vi "ADIS16470 IMU Example.vi"() -> ()   [LabVIEW 2019]
uses:
  <vilib>/Utility/RT CPU Load.ctl
  ADIS16470Lib/Typedef/ADIS16470 Hardware Configuration.ctl
  <vilib>/Rock Robotics/WPI/SPI/WPI_SPIMode.ctl
  <vilib>/Rock Robotics/SystemInterfaces/DIO/FPGA_DIOChannel.ctl
  <vilib>/Rock Robotics/SystemInterfaces/spilib/spi_bus.ctl
  <vilib>/NI_Real-Time Target Support.lvlib
panel:
  in  "Reset?":bool
  out "Integrated Gyro Angle":T1(graph)
  out "Calibrated?":bool
  out "Ready?":bool
  in  "Hardware Config":T2={"SPI Clock Rate (Hz)"=2000000.0, "IMU SPI Mode (3)"=enum."Mode 3 (Clk Idle High,Sample on Trailing)", "IMU Reset Pin"=enum."SPI Port CS2", "IMU SPI Bus"=enum."SPI On-Board, CS0", "IMU Data Ready Pin"=enum."SPI Port CS1", "Stall Config"={"Pow2BytesPerRead"=1, "StallTicks"=1000, "CsToSclkTicks"=5}}
  out "CPU loads":T6[](array[typedef]) {"ISR (%)" format="%#.2f"; "Idle (%)" format="%#.2f"; "Background (%)" format="%#.2f"; "Normal (%)" format="%#.2f"; "Above Normal (%)" format="%#.2f"; "High (%)" format="%#.2g"; "Timed Structures (%)" format="%#.2g"; "Time Critical (%)" format="%#.2g"; "Total (%)" format="%#.2g"}
  in  "stop":bool
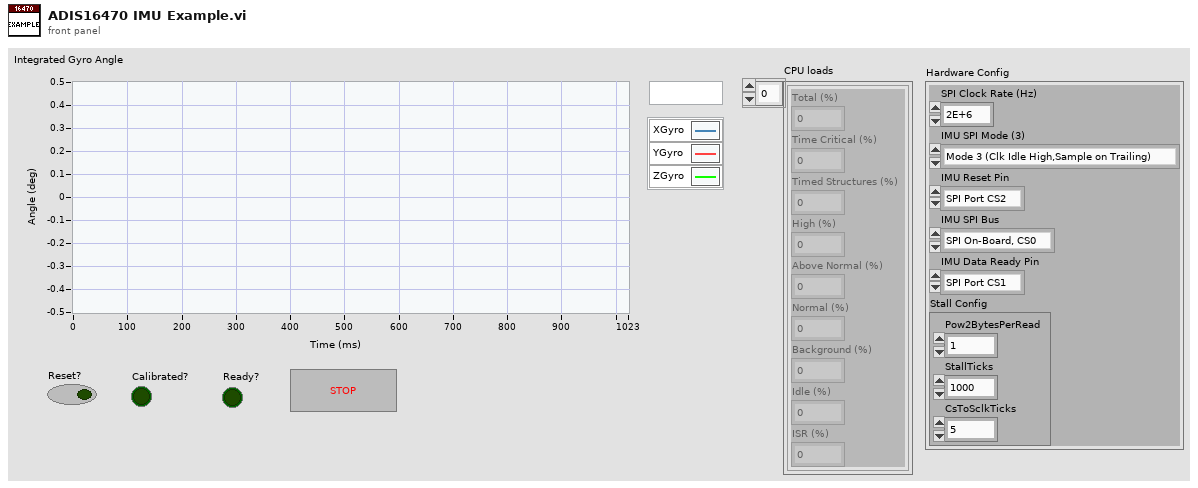
[diagram p1: front panel]
types:
  T1 = cluster{"XAngle":dbl, "YAngle":dbl, "ZAngle":dbl}
  T2 = typedef "ADIS16470 Hardware Configuration.ctl" = cluster{"SPI Clock Rate (Hz)":dbl, "IMU SPI Mode (3)":T3, "IMU Reset Pin":T4, "IMU SPI Bus":T5, "IMU Data Ready Pin":T4, "Stall Config":cluster{"Pow2BytesPerRead":u8, "StallTicks":u16, "CsToSclkTicks":u8}}
  T3 = typedef "WPI_SPIMode.ctl" = enum16{"Mode 0 (Clk Idle Low,Sample on Leading)", "Mode 1 (Clk Idle Low,Sample on Trailing)", "Mode 2 (Clk Idle High,Sample on Leading)", "Mode 3 (Clk Idle High,Sample on Trailing)"}
  T4 = typedef "FPGA_DIOChannel.ctl" = enum8{"DIO 0", "DIO 1", "DIO 2", "DIO 3", "DIO 4", "DIO 5", "DIO 6", "DIO 7", "DIO 8", "DIO 9", "DIO MXP 0", "DIO MXP 1", "DIO MXP 2", "DIO MXP 3", "DIO MXP 4", "DIO MXP 5", "DIO MXP 6", "DIO MXP 7", "DIO MXP 8", "DIO MXP 9", "DIO MXP 10", "DIO MXP 11", "DIO MXP 12", "DIO MXP 13", "DIO MXP 14", "DIO MXP 15", "SPI Port CS1", "SPI Port CS2", "SPI Port CS3", "SPI Port MISO", "SPI Port MOSI", "Invalid"}
  T5 = typedef "spi_bus.ctl" = enum16{"SPI On-Board, CS0", "SPI On-Board, CS1", "SPI On-Board, CS2", "SPI On-Board, CS3", "SPI MXP", "Invalid"}
  T6 = typedef "NI_Real-Time Target Support.lvlib/RT CPU Load.ctl" = cluster{"Total (%)":dbl, "Time Critical (%)":dbl, "Timed Structures (%)":dbl, "High (%)":dbl, "Above Normal (%)":dbl, "Normal (%)":dbl, "Background (%)":dbl, "Idle (%)":dbl, "ISR (%)":dbl}
  T7 = typedef "ADIS16470 Device Reference.ctl" = cluster{"DevStatus":errorcluster, "Hardware Config":T2, "End Calibration":refnum<notifier>, "Calibration Complete":refnum<notifier>, "Status FIFO":refnum<k33>, "Last Value Reference":refnum<data-value>, "Sychronous Process VI":T8, "Cmd FIFO":refnum<k33>, "Source":T9, "Data FIFO":refnum<k33>}
  T8 = typedef "ADIS16470 Process.ctl" = refnum<vi>
  T9 = typedef "FPGA_CounterEncoderSourceConvertionLVSourceType.ctl" = cluster{"DevStatus":errorcluster, "AnalogTriggerMode?":bool, "DigitalMode":cluster{"DIO Channel":T10}, "AnalogTriggerMode":cluster{"AnalogTriggerIndex":T11, "OutputType":T12}}
  T10 = typedef "FPGA_DIODigitalSourceChannel.ctl" = enum8{"DIO 0", "DIO 1", "DIO 2", "DIO 3", "DIO 4", "DIO 5", "DIO 6", "DIO 7", "DIO 8", "DIO 9", "DIO MXP 0", "DIO MXP 1", "DIO MXP 2", "DIO MXP 3", "DIO MXP 4", "DIO MXP 5", "DIO MXP 6", "DIO MXP 7", "DIO MXP 8", "DIO MXP 9", "DIO MXP 10", "DIO MXP 11", "DIO MXP 12", "DIO MXP 13", "DIO MXP 14", "DIO MXP 15", "SPI Port CS1", "SPI Port CS2", "SPI Port CS3", "SPI Port MISO", "SPI Port MOSI", "Disabled"}
  T11 = typedef "FPGA_AnalogTriggerIndex.ctl" = enum8{"Trig 0", "Trig 1", "Trig 2", "Trig 3", "Trig 4", "Trig 5", "Trig 6", "Trig 7", "Invalid"}
  T12 = typedef "FPGA_AnalogTriggerOutType.ctl" = enum16{"InWindow", "TriggerState", "Rising", "Falling"}
  T13 = typedef "ADIS16470 Status.ctl" = cluster{"Calibrated?":bool}
  T14 = typedef "ADIS16470 Data.ctl" = cluster{"XAngle":dbl, "YAngle":dbl, "ZAngle":dbl}
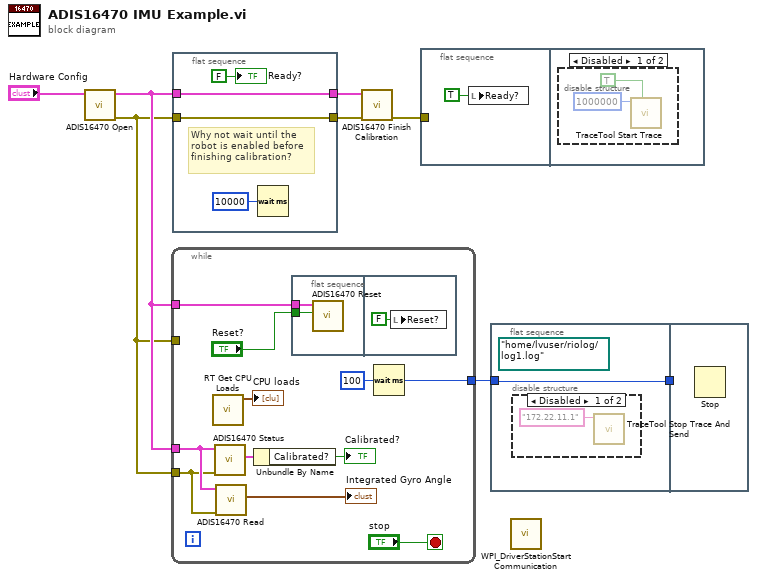
[diagram p0: block diagram]
diagram:
  n1 = call "ADIS16470 Open.vi"("Hardware Config"="Hardware Config") -> ("error out"=w2:errorcluster, "ADIS16470DevRef"=w3:T7)  [unwired: 9 in]
  n2 = while {
    tunnel: [w16] -> w8
    tunnel: w3 -> [w13]
    tunnel: w2 -> [w12]
    tunnel: w3 -> [w10]
    tunnel: w2 -> [_]
    stop <- "stop" stop-if-true
    n3 = call <vilib>:"RT Get CPU Loads.vi"() -> ("CPU loads"=→"CPU loads":T6[])  [unwired: 10 in, 1 out]
    n4 = call "ADIS16470 Status.vi"("error in (no error)"=w12, "ADIS16470DevRef"=w13) -> ("ADIS16470 Status"=w14:T13)  [unwired: 7 in, 2 out]
    n5 = call "ADIS16470 Read.vi"("error in (no error)"=w12, "ADIS16470DevRef"=w13) -> ("ADIS16470 Value"=→"Integrated Gyro Angle":T14)  [unwired: 6 in, 3 out]
    n6 = Unbundle By Name(w14) -> ("Calibrated?"=→"Calibrated?":bool)
    n7 = flat-sequence {
      tunnel: "Reset?" -> [w21]
      tunnel: w10 -> [w20]
      frame #0 {
        n8 = call "ADIS16470 Reset.vi"("Reset?"=w21, "ADIS16470DevRef"=w20) -> ()  [unwired: 8 in, 2 out]
      }
      frame #1 {
        n9 = local write "Reset?"(FALSE ("Reset?")) -> ()
      }
    }
    n10 = Wait (ms)(milliseconds to wait=u32 100) -> (millisecond timer value=w16:u32)
  }
  n11 = flat-sequence {
    tunnel: w3 -> [w24]
    tunnel: [w24] -> w6
    tunnel: w2 -> [w23]
    tunnel: [w23] -> w5
    frame #0 {
      # "Why not wait until the \nrobot is enabled before\nfinishing calibration?"
      n12 = Wait (ms)(milliseconds to wait=u32 10000) -> ()  [unwired: 1 out]
      "Ready?" <- FALSE ("Ready?")
    }
  }
  n13 = call "ADIS16470 Finish Calibration.vi"("error in (no error)"=w5, "ADIS16470DevRef in"=w6) -> ("error out"=w4:errorcluster)  [unwired: 8 in, 1 out]
  n14 = flat-sequence {
    tunnel: w4 -> [_]
    frame #0 {
      n15 = local write "Ready?"(TRUE ("Ready?")) -> ()
    }
    frame #1 {
      n16 = disable-structure shown="Disabled" {
        frame Disabled {
          n17 = call <vilib>:"TraceTool Start Trace.vi"("Detailed Tracing? (F)"=TRUE, "Buffer Size (250000 bytes)"=1000000) -> ()  [unwired: 8 in, 2 out]
        }
        frame Enabled {
        }
      }
    }
  }
  n18 = flat-sequence {
    tunnel: w8 -> [w30]
    tunnel: [w30] -> w1
    tunnel: w1 -> [_]
    frame #0 {
      (unwired) path "/home/lvuser/riolog/log1.log" ("Path to Trace Log")
      n19 = disable-structure shown="Disabled" {
        frame Disabled {
          n20 = call <vilib>:"TraceTool Stop Trace And Send.vi"("Trace Host Network Address"="172.22.11.1") -> ()  [unwired: 10 in, 1 out]
        }
        frame Enabled {
        }
      }
    }
    frame #1 {
      n21 = Stop() -> ()  [unwired: 1 in]
    }
  }
  n22 = call <vilib>:"WPI_DriverStationStart Communication.vi"() -> ()  [unwired: 12 in]
